vi "Config Type.vi"(11 "Time Condition in":refnum<class "Time Condition.lvclass">) -> (2 "Condition Config":refnum<class "Condition Config.lvclass">)   [LabVIEW 2020, in "VolatusSeq.lvlib" / "Time Condition.lvclass"]
uses:
  Time Condition.lvclass
  Time Condition.lvclass/Time Condition.ctl
  VolatusSeqConfig/Time Condition Config/Time Condition Config.lvclass
  C:/dev/lv20CE/relink/lv-volatus/VolatusSeqConfig/Condition Config/Condition Config.lvclass
  C:/dev/lv20CE/relink/lv-volatus/VolatusSeqConfig/Time Condition Config/Time Condition Config.lvclass
  VolatusSeqConfig/Condition Config/Condition Config.lvclass
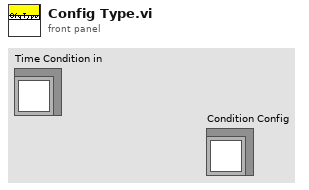
[diagram p1: front panel]
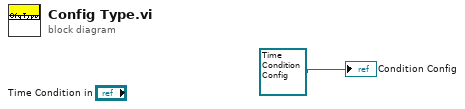
[diagram p0: block diagram]
diagram:
  "Condition Config" <- refnum<class "Time Condition Config.lvclass"> refnum ("VolatusSeqConfig.lvlib:Time Condition Config.lvclass")
